vi "subFilterForExporters.vi"(8 "error in (no error)":errorcluster, 9 "Addons":path[](array[path]), 11 "UIManager in":refnum<class "UIManager.lvclass">) -> (0 "error out":errorcluster, 3 "UIManager out":refnum<class "UIManager.lvclass">)   [LabVIEW 2020, in "DependencyInspector.lvlib" / "UIManager.lvclass"]
uses:
  UIManager.lvclass
  UIManager.lvclass/UIManager.ctl
  obj/Addons/ExtensionInterfaces.lvlibp/IExporter/IExporter.lvclass
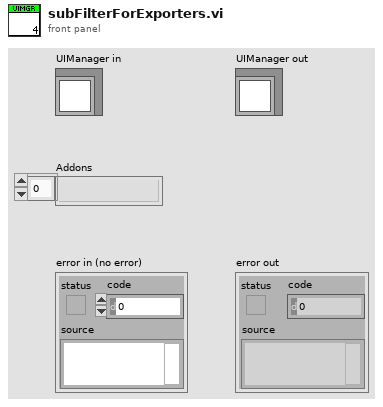
[diagram p1: front panel]
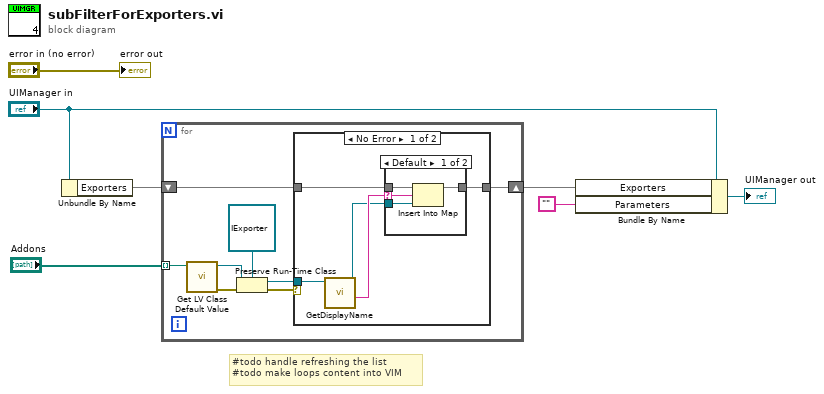
[diagram p0: block diagram]
diagram:
  # "#todo handle refreshing the list\n#todo make loops content into VIM"
  n1 = Unbundle By Name("UIManager in") -> ("Exporters"=w1:map{string, refnum<class "IExporter.lvclass">})
  n2 = for {
    tunnel: "Addons" -> [w15] mode=indexing
    shift-right: [w9] -> w6
    shift-left: w1 -> [w11]
    n3 = call <vilib>:"Get LV Class Default Value.vi"("class path"=w15) -> ("error out"=w14:errorcluster, "object"=w13:refnum<class>)  [unwired: 9 in]
    n4 = Preserve Run-Time Class(object in=w13, error in=w14, 2:refnum<class "IExporter.lvclass"> refnum ("ExtensionInterfaces.lvlibp:IExporter.lvclass")) -> (object out=w10:refnum<class "IExporter.lvclass">, error out=w12:errorcluster)
    n5 = case shown="No Error" w12 {
      tunnel: w11 -> [w19 w26]
      tunnel: w10 -> [w20 _]
      tunnel: [w16 w26] -> w9
      frame No Error {
        n6 = call-dynamic "GetDisplayName.vi"("IExporter in"=w20) -> ("Display name"=w18:string, "IExporter out"=w17:refnum<class "IExporter.lvclass">)  [unwired: 8 in, 1 out]
        n7 = case shown="Default" w18 {
          selector: w18 -> [w21 _]
          tunnel: w19 -> [w24 w25]
          tunnel: w17 -> [w23 _]
          tunnel: [w22 w25] -> w16
          frame Default {
            n8 = Insert Into Map(map in=w24, key=w21, value=w23) -> (map out=w22:map{string, refnum<class "IExporter.lvclass">})  [unwired: 2 out]
          }
          frame "" {
          }
        }
      }
      frame Error {
      }
    }
  }
  n9 = Bundle By Name(cluster="UIManager in", "Exporters"=w6, "Parameters"="") -> (→"UIManager out":refnum<class "UIManager.lvclass">)
  "error out" <- "error in (no error)"
